vi "Creating an Event Structure.vi"() -> ()   [LabVIEW 2015]
panel:
  out "Numeric Out":dbl
  in  "Numeric In":dbl
  out "Boolean":bool
  out "Current Time":timestamp format="%<%x %X>T"
  in  "Stop":bool
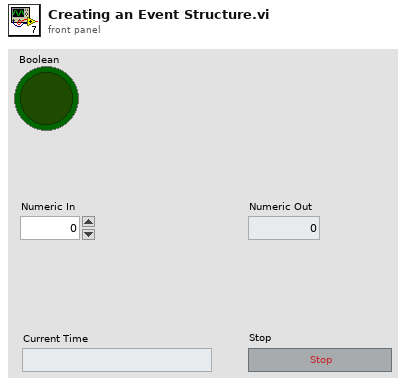
[diagram p1: front panel]
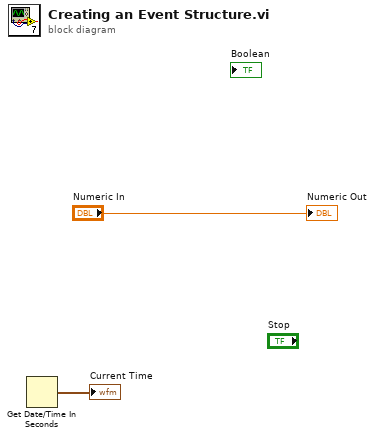
[diagram p0: block diagram]
diagram:
  n1 = Get Date/Time In Seconds() -> (seconds since 1Jan1904=→"Current Time":timestamp)
  "Numeric Out" <- "Numeric In"
